vi "OMRON_HostLink协议通讯.vi"(0 "串口输入":refnum<visa-resource-name>, 1 "FCS校验码":string, 5 "写入数据（读）":string="@00RD00000002", 7 "读写方式":bool, 9 "写入数据（写）":string="@00WD000000010002", 11 "错误输入（无错误）":errorcluster) -> (4 "串口输出":refnum<visa-resource-name>, 10 "通讯数据":string, 15 "错误输出":errorcluster)   [LabVIEW 2014]
panel:
  # "串口参数：\n波特率：9600\n数据位：7\n停止位：2\n校验位：偶校验（EVEN）"
  # "默认为读（F）"
  # "通讯格式说明：\n   发送：\n     读：          起始符        节点号                 命令码        开始字             字数         FCS校验码   终止符\n                        @              00                       RD          0000              0002                \n起始符：必须以@开始\n节点号：默认是00，由DM6648和DM6653指定\n命令码：RD（DM数据区读）\n开始字：0000（个人理解是起始地址）（10进制数据）\n字数：0002（要读取的字的个数）（10进制数据）\nFCS校验码：\n终止符：*CR（由*和回车组成）（一定要组合，一次最多字符长度是131超过之后利用的是分隔符来读取的）\n     写：          起始符        节点号           命令码        开始字        第一个数据（字）  第二个数据（字）      FCS校验码    终止符\n                        @              00                WD          0000              0001                    0010\n起始符：必须以@开始\n节点号：默认是00，由DM6648和DM6653指定\n命令码：WD（DM数据区写）\n开始字：0000（个人理解是起始地址）（10进制数据）\n第一/二个数据（字）：0001/0010（写入的数据1和16）（16进制数据）\nFCS校验码：\n终止符：*CR（由*和回车组成）（一定要组合，一次最多字符长度是131超过之后利用的是分隔符来读取的）"
  # "通讯格式说明：\n   接收：\n     读：          起始符        节点号           命令码          尾码      第一个数据（字）  第二个数据（字）      FCS校验码    终止符\n                        @              00                RD             00              0001                0010\n起始符：必须以@开始\n节点号：默认是00，由DM6648和DM6653指定\n命令码：RD（DM数据区读）\n尾码：00（正确完成）\n第一/二个数据（字）：0001/0010（读取的数据1和16）（16进制数据）\nFCS校验码：\n终止符：*CR（由*和回车组成）（一定要组合，一次最多字符长度是131超过之后利用的是分隔符来读取的）\n    写：          起始符        节点号          命令码        尾码      FCS校验码    终止符          \n                       @              00              WD           00              \n起始符：必须以@开始\n节点号：默认是00，由DM6648和DM6653指定\n命令码：WD（DM数据区写）\n尾码：00（正确完成）\nFCS校验码：\n终止符：*CR（由*和回车组成）（一定要组合，一次最多字符长度是131超过之后利用的是分隔符来读取的）"
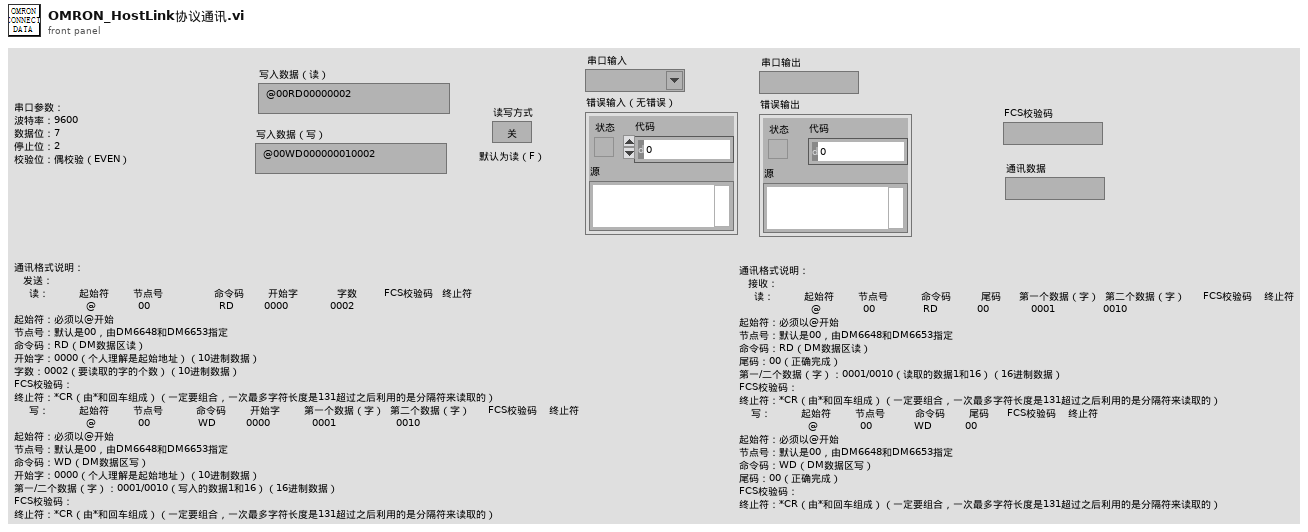
[diagram p1: front panel]
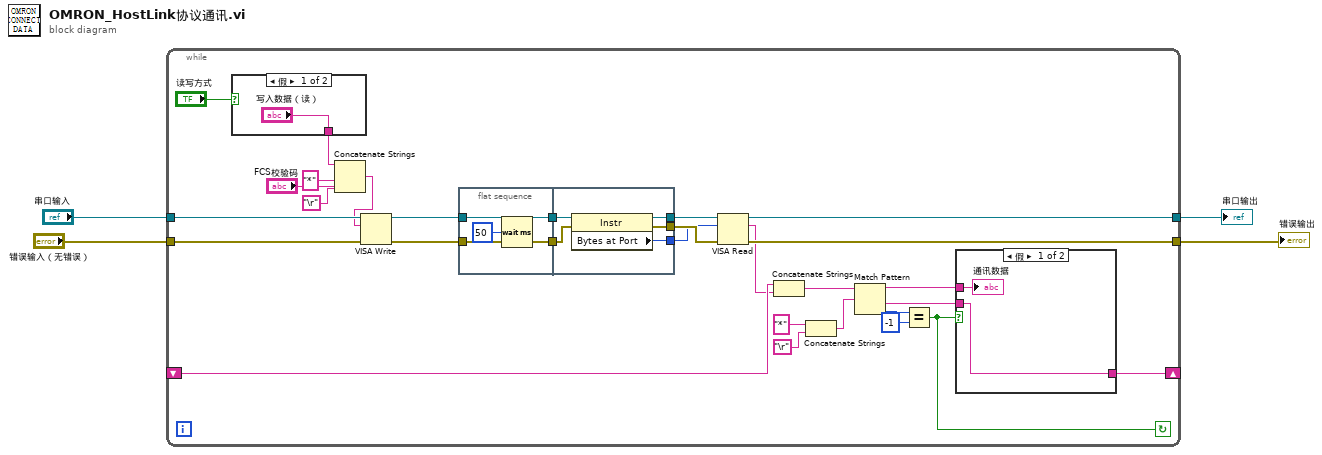
[diagram p0: block diagram]
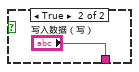
[diagram p2: hidden frame]
diagram:
  n1 = while {
    tunnel: "串口输入" -> [w31]
    tunnel: "错误输入（无错误）" -> [w30]
    tunnel: [w24] -> w2
    tunnel: [w23] -> w1
    shift-right: [w13] -> _
    shift-left: _ -> [w22]
    stop <- w11 continue-if-true
    n2 = case shown="假" "读写方式" {
      tunnel: ["写入数据（读）" "写入数据（写）"] -> w8
      frame False {
      }
      frame True {
      }
    }
    n3 = Concatenate Strings(w8, "FCS校验码", "*" ("搜索字符串"), "\r") -> (w6:string)
    n4 = VISA Write(VISA resource name=w31, write buffer=w6, error in (no error)=w30) -> (VISA resource name out=w29:refnum<visa-resource-name>, error out=w28:errorcluster)  [unwired: 1 out]
    n5 = flat-sequence {
      tunnel: [w40] -> w33
      tunnel: w29 -> [w40]
      tunnel: w28 -> [w39]
      tunnel: [w39] -> w32
      tunnel: w33 -> [w46]
      tunnel: w32 -> [w45]
      tunnel: [w44] -> w27
      tunnel: [w43] -> w26
      tunnel: [w42] -> w25
      frame #0 {
        n6 = Wait (ms)(milliseconds to wait=u32 50 ("等待时间（毫秒）")) -> ()  [unwired: 1 out]
      }
      frame #1 {
        n7 = property class="Instr"(reference=w46, error in=w45) -> (reference out=w44:refnum<visa-resource-name>, error out=w43:errorcluster, "Bytes at Port"=w42:u32)
      }
    }
    n8 = VISA Read(VISA resource name=w27, byte count=w25, error in (no error)=w26) -> (VISA resource name out=w24:refnum<visa-resource-name>, read buffer=w21:string, error out=w23:errorcluster)  [unwired: 1 out]
    n9 = Concatenate Strings(w22, w21) -> (w20:string)
    n10 = Concatenate Strings("*" ("搜索字符串"), "\r") -> (w17:string)
    n11 = Match Pattern(string=w20, regular expression=w17) -> (before substring=w14:string, after substring=w12:string, offset past match=w15:i32)  [unwired: 1 in, 1 out]
    n12 = Equal?(x=w15, y=-1) -> (x = y?=w11:bool)
    n13 = case shown="假" w11 {
      tunnel: w14 -> [w36 w38]
      tunnel: [w37 w38] -> w13
      tunnel: w12 -> [w37 _]
      frame False {
        "通讯数据" <- w36
      }
      frame True {
      }
    }
  }
  "串口输出" <- w2
  "错误输出" <- w1
